vi "readCNT.vi"(8 "error in (no error)":errorcluster) -> (0 "error out":errorcluster, 2 "medicion":dbl)   [LabVIEW 2019, in "CNT90_GPIB.lvlib"]
uses:
  CNT90_GPIB.lvlib
panel:
  out "read buffer":string
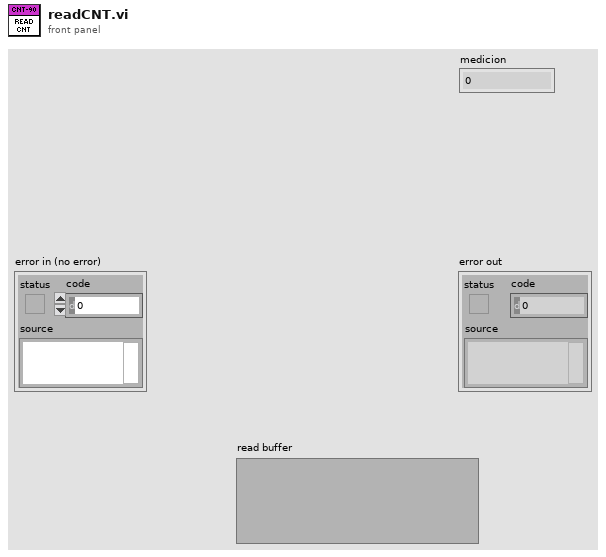
[diagram p1: front panel]
types:
  T1 = cluster{"error":bool, "code":i32, "source":string}
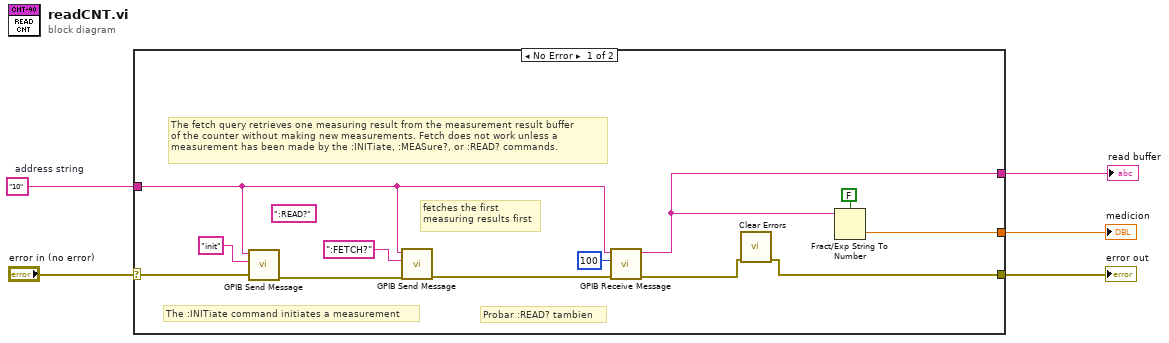
[diagram p0: block diagram]
diagram:
  w3 = "10"  # address string
  n1 = case shown="No Error" "error in (no error)" {
    selector: "error in (no error)" -> [w13 w18]
    tunnel: [w8 w18] -> w4
    tunnel: w3 -> [w12 _]
    tunnel: [w11 _] -> w2
    tunnel: [w10 _] -> w1
    frame No Error {
      (unwired) ":READ?" ("write buffer")
      # "Probar :READ? tambien"
      # "The :INITiate command initiates a measurement"
      # "The fetch query retrieves one measuring result from the measurement result buffer\nof the counter without making new measurements. Fetch does not work unless a\nmeasurement has been made by the :INITiate, :MEASure?, or :READ? commands."
      # "fetches the first\nmeasuring results first"
      n2 = call <instrlib>:"GPIB Send Message.vi"("address string"=w12, "write buffer"="init", "error in"=w13) -> ("error out"=w16:T1)  [unwired: 4 in, 2 out]
      n3 = call <instrlib>:"GPIB Send Message.vi"("address string"=w12, "write buffer"=":FETCH?", "error in"=w16) -> ("error out"=w14:T1)  [unwired: 4 in, 2 out]
      n4 = call <instrlib>:"GPIB Receive Message.vi"("address string"=w12, "byte count"=100, "error in"=w14) -> ("read buffer"=w10:string, "error out"=w9:T1)  [unwired: 4 in, 1 out]
      n5 = call <vilib>:"Clear Errors.vi"("error in (no error)"=w9) -> ("error out"=w8:errorcluster)  [unwired: 5 in, 1 out]
      n6 = Fract/Exp String To Number(use system decimal point (T)=FALSE, string=w10) -> (number=w11:dbl)  [unwired: 2 in, 1 out]
    }
    frame Error {
    }
  }
  "error out" <- w4
  "medicion" <- w2
  "read buffer" <- w1
